vi "CRYMake Command Idx.vi"() -> (3 "New Command Idx":i32)   [LabVIEW 2013]
uses:
  CRYNew View Global.vi
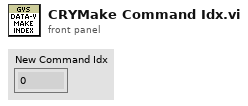
[diagram p1: front panel]
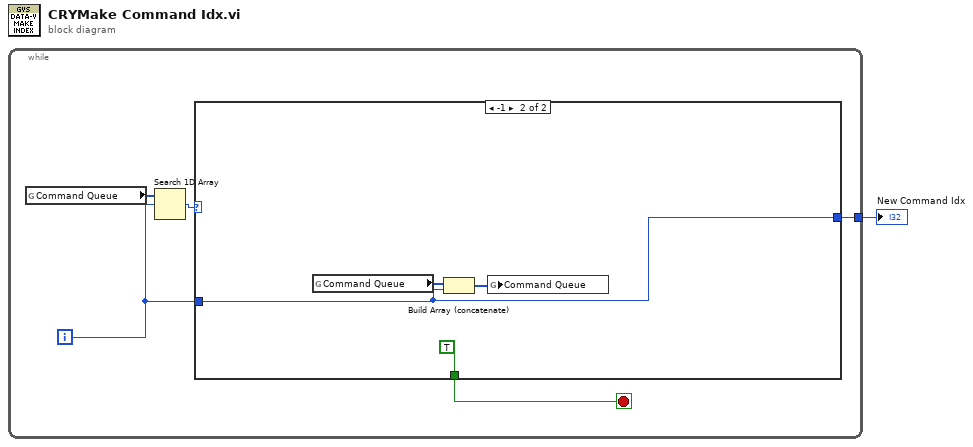
[diagram p0: block diagram]
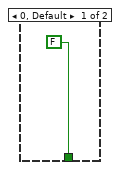
[diagram p2: hidden frame]
diagram:
  n1 = while {
    tunnel: [w3] -> w1
    i -> [w2]
    stop <- w4 stop-if-true
    n2 = global read "CRYNew View Global.vi" "Command Queue"() -> (w6:i32[])
    n3 = Search 1D Array(1D array=w6, element=w2) -> (index of element=w5:i32)  [unwired: 1 in]
    n4 = case shown="-1" w5 {
      tunnel: w2 -> [_ w8]
      tunnel: [FALSE TRUE] -> w4
      tunnel: [_ w8] -> w3
      frame 0, Default {
      }
      frame -1 {
        n5 = global read "CRYNew View Global.vi" "Command Queue"() -> (w11:i32[])
        n6 = Build Array (concatenate)(w11, w8) -> (w10:i32[])
        n7 = global write "CRYNew View Global.vi" "Command Queue"(w10) -> ()
      }
    }
  }
  "New Command Idx" <- w1
